vi "CAN Get Msg.vi"(10 "CANIndex":u8, 11 "DevIndex":i32) -> (2 "function return":i32, 3 "pCanGetMsg":T1)   [LabVIEW 2010, in "usb2can.lvlib"]
doc: "int WINAPI CAN_GetMsg(int DevIndex, unsigned char CANIndex, PCAN_MSG pCanGetMsg);"
uses:
  usb2can.lvlib
  USB2XXX.dll
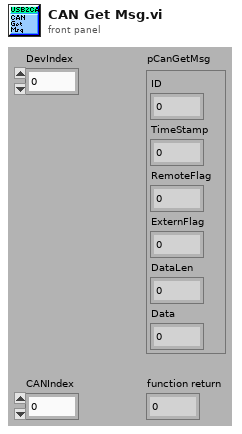
[diagram p1: front panel]
types:
  T1 = cluster{"ID":u32, "TimeStamp":u32, "RemoteFlag":u8, "ExternFlag":u8, "DataLen":u8, "Data":u8}
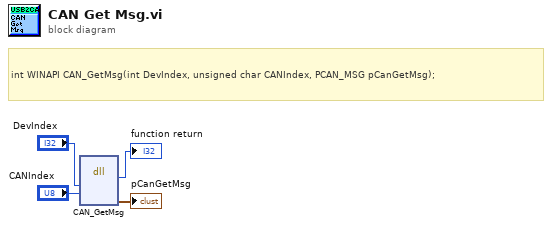
[diagram p0: block diagram]
diagram:
  # "int WINAPI CAN_GetMsg(int DevIndex, unsigned char CANIndex, PCAN_MSG pCanGetMsg);"
  n1 = dll-call lib="F:/OtherWork/STM32/USB2XXX_Example/trunk/Labview/PublicFiles/usb2can/USB2XXX.*" fn="CAN_GetMsg"("DevIndex"="DevIndex", "CANIndex"="CANIndex") -> (→"function return":i32, "pCanGetMsg"=→"pCanGetMsg":T1)  [unwired: 6 in, 2 out]
